vi "VPA QC XDCR DAQ.vi"(8 "error in (no error)":errorcluster, 9 "task/channels in":refnum<k21>, 10 "DAQ Ref Cluster":T1) -> (0 "error out":errorcluster, 2 "DAQ Ref Cluster Out":T1)   [LabVIEW 2013]
uses:
  Controls/VPA QC DAQ Ref Cluster.ctl
  <vilib>/DAQmx/read.llb/DAQmx Read (Analog 1D DBL 1Chan NSamp).vi
  <vilib>/DAQmx/miscellaneous.llb/DAQmx Fill In Error Info.vi
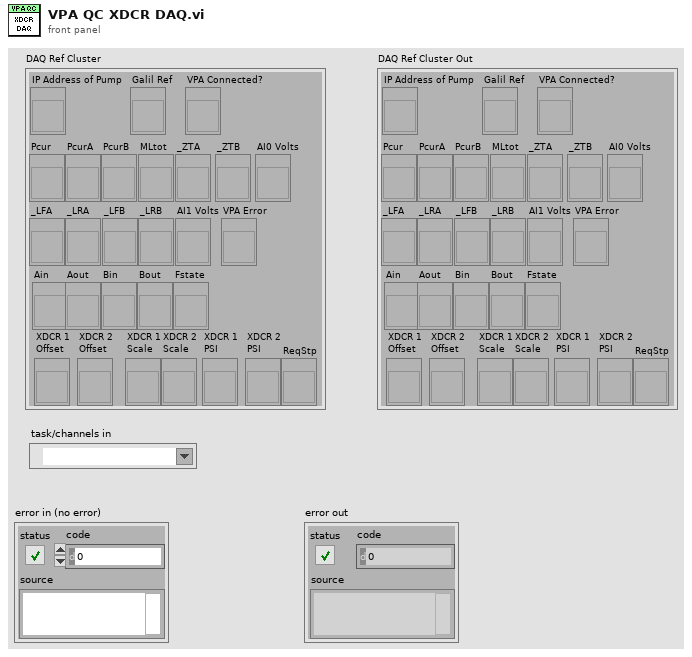
[diagram p1: front panel]
types:
  T1 = typedef "VPA QC DAQ Ref Cluster.ctl" = cluster{"IP Address of Pump":refnum<vi>, "Galil Ref":refnum<vi>, "VPA Connected?":refnum<vi>, "Pcur":refnum<vi>, "PcurA":refnum<vi>, "PcurB":refnum<vi>, "MLtot":refnum<vi>, "_LFA":refnum<vi>, "_LRA":refnum<vi>, "_LFB":refnum<vi>, "_LRB":refnum<vi>, "_ZTA":refnum<vi>, "_ZTB":refnum<vi>, "AI0 Volts":refnum<vi>, "AI1 Volts":refnum<vi>, "VPA Error":refnum<vi>, "Ain":refnum<vi>, "Aout":refnum<vi>, "Bin":refnum<vi>, "Bout":refnum<vi>, "Fstate":refnum<vi>, "XDCR 1\nOffset":refnum<vi>, "XDCR 2 \nOffset":refnum<vi>, "XDCR 1\nScale":refnum<vi>, "XDCR 2\nScale":refnum<vi>, "XDCR 1\nPSI":refnum<vi>, "XDCR 2\nPSI":refnum<vi>, "ReqStp":refnum<vi>}
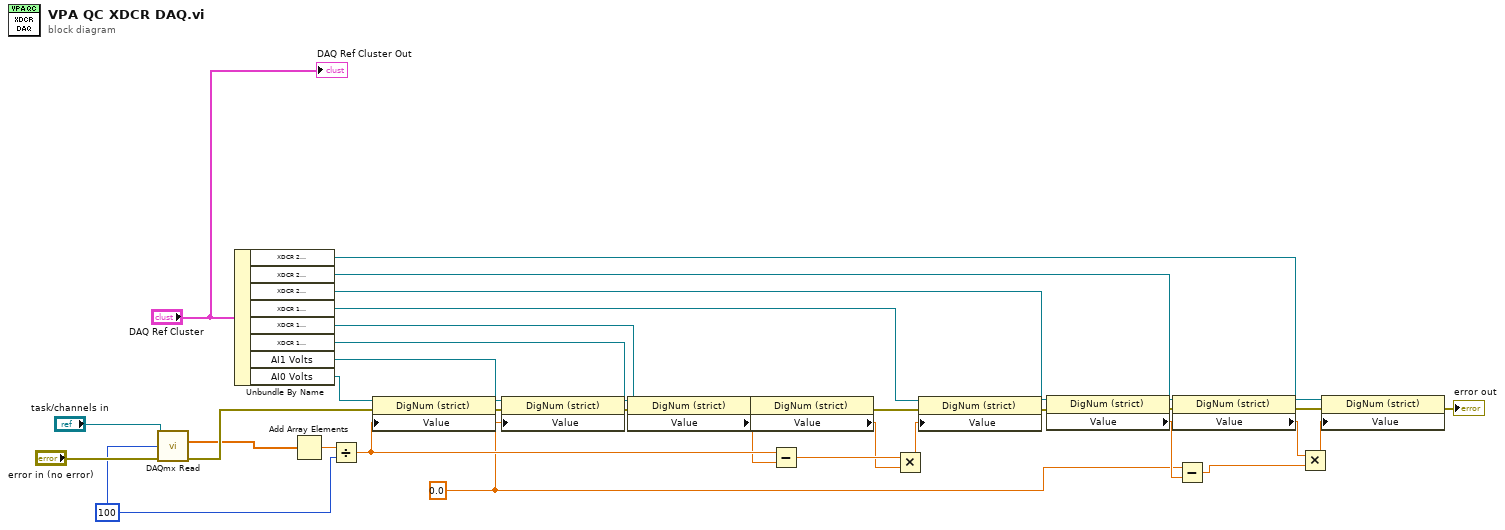
[diagram p0: block diagram]
diagram:
  w2 = 0.0 ("Value")
  w1 = 100 ("number of samples per channel")
  n1 = call-poly <vilib>:"DAQmx Read.vi"("task/channels in"="task/channels in", "number of samples per channel"=w1, "error in"="error in (no error)") -> ("data"=w3:dbl[], "error out"=w27:errorcluster)  [unwired: 10 in, 1 out]
  n2 = Unbundle By Name("DAQ Ref Cluster") -> ("XDCR 2\nPSI"=w12:refnum<vi>, "XDCR 2\nScale"=w18:refnum<vi>, "XDCR 2 \nOffset"=w19:refnum<vi>, "XDCR 1\nPSI"=w21:refnum<vi>, "XDCR 1\nScale"=w23:refnum<vi>, "XDCR 1\nOffset"=w26:refnum<vi>, "AI1 Volts"=w29:refnum<vi>, "AI0 Volts"=w30:refnum<vi>)
  n3 = Add Array Elements(numeric array=w3) -> (sum=w33:dbl)
  n4 = Divide(x=w33, y=w1) -> (x/y=w25:dbl)
  n5 = property class="DigNum (strict)"(reference=w30, error in=w27, "Value"=w25) -> (error out=w28:errorcluster)  [unwired: 1 out]
  n6 = property class="DigNum (strict)"(reference=w29, error in=w28, "Value"=w2) -> (error out=w17:errorcluster)  [unwired: 1 out]
  n7 = property class="DigNum (strict)"(reference=w26, error in=w17) -> (error out=w16:errorcluster, "Value"=w24:dbl)  [unwired: 1 out]
  n8 = property class="DigNum (strict)"(reference=w23, error in=w16) -> (error out=w15:errorcluster, "Value"=w22:dbl)  [unwired: 1 out]
  n9 = Subtract(x=w25, y=w24) -> (x-y=w32:dbl)
  n10 = Multiply(x=w32, y=w22) -> (x*y=w20:dbl)
  n11 = property class="DigNum (strict)"(reference=w21, error in=w15, "Value"=w20) -> (error out=w14:errorcluster)  [unwired: 1 out]
  n12 = property class="DigNum (strict)"(reference=w19, error in=w14) -> (error out=w13:errorcluster, "Value"=w11:dbl)  [unwired: 1 out]
  n13 = property class="DigNum (strict)"(reference=w18, error in=w13) -> (error out=w6:errorcluster, "Value"=w10:dbl)  [unwired: 1 out]
  n14 = Subtract(x=w2, y=w11) -> (x-y=w9:dbl)
  n15 = Multiply(x=w10, y=w9) -> (x*y=w8:dbl)
  n16 = property class="DigNum (strict)"(reference=w12, error in=w6, "Value"=w8) -> (error out=→"error out":errorcluster)  [unwired: 1 out]
  "DAQ Ref Cluster Out" <- "DAQ Ref Cluster"
